vi "Raycaster_DrawSubBuffer.vi"(5 "Sub Buffer":u8, 7 "Num Columns":i16=100, 8 "Wall Height In":i16[](array[numeric]), 9 "Buffer In":u8[](array[numeric]), 10 "Game State":T1, 11 "Camera X":fxp<+/-,32,16>[](array[numeric])) -> (0 "Wall Height Out":i16[](array[numeric]), 1 "Buffer Out":u8[](array[numeric]))   [LabVIEW 2020]
uses:
  Controls/Game_State.ctl
  Controls/Player_LocationInfo.ctl
  Controls/Player_LocationInfoAxis.ctl
  Controls/Map_Position.ctl
  Controls/Raycaster_DDACalcs.ctl
  Controls/Raycaster_WallColumnAxis.ctl
  Math_FXPtoI16.vi
  Math_Multiply_FXP.vi
  Math_Add_FXP.vi
  Math_Reciprocal.vi
  Math_Subtract_FXP.vi
  Globals/MAP_DIM.vi
  Map_ReadValue.vi
  Math_Divide_FXP.vi
  Globals/HEIGHT_DIV_2.vi
  Map_GetMaps.vi
  Globals/FGV_TileVisible.vi
  <vilib>/Utility/file.llb/Application Directory.vi
  <vilib>/rvi/DataTransferAndStorage/Container/XNode/niFpgaContainer.xnode
  <vilib>/rvi/Memory/Memory_Emulation/nirvimemoryEmulation.vi
  <vilib>/rvi/Memory/Memory_Emulation/nirvimemoryFastEmulation.vi
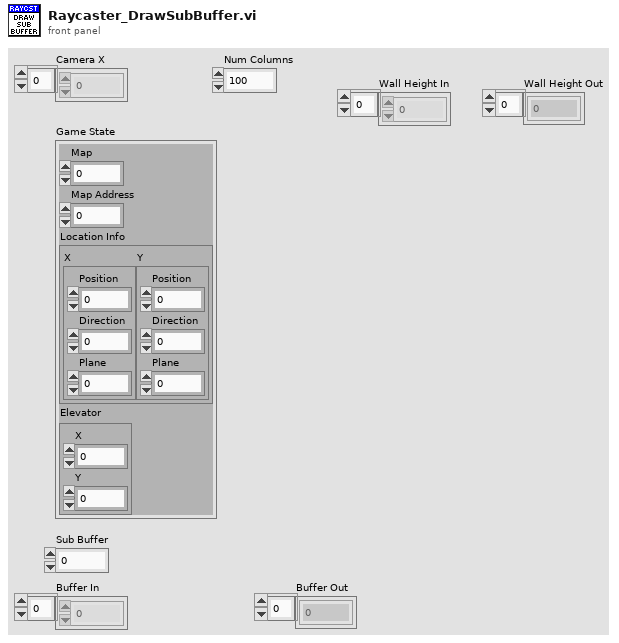
[diagram p1: front panel]
types:
  T1 = typedef "Game_State.ctl" = cluster{"Map":u8, "Map Address":u32, "Location Info":T2, "Elevator":T4}
  T2 = typedef "Player_LocationInfo.ctl" = cluster{"X":T3, "Y":T3}
  T3 = typedef "Player_LocationInfoAxis.ctl" = cluster{"Position":fxp<+/-,32,16>, "Direction":fxp<+/-,32,16>, "Plane":fxp<+/-,32,16>}
  T4 = typedef "Map_Position.ctl" = cluster{"X":fxp<+/-,32,16>, "Y":fxp<+/-,32,16>}
  T5 = typedef "Raycaster_DDACalcs.ctl" = cluster{"X":T6, "Y":T6, "Side":u8, "Perp Wall Distance":fxp<+/-,32,16>, "Wall Collision":u8}
  T6 = typedef "Raycaster_WallColumnAxis.ctl" = cluster{"Ray Direction":fxp<+/-,32,16>, "Side Distance":fxp<+/-,32,16>, "Delta Distance":fxp<+/-,32,16>, "Step":i16, "Map":i16}
  T7 = typedef "Raycaster_ScreenCalcs.ctl" = cluster{"Length":i16, "Pixel Start":i16, "Pixel End":i16, "Draw Start":i16}
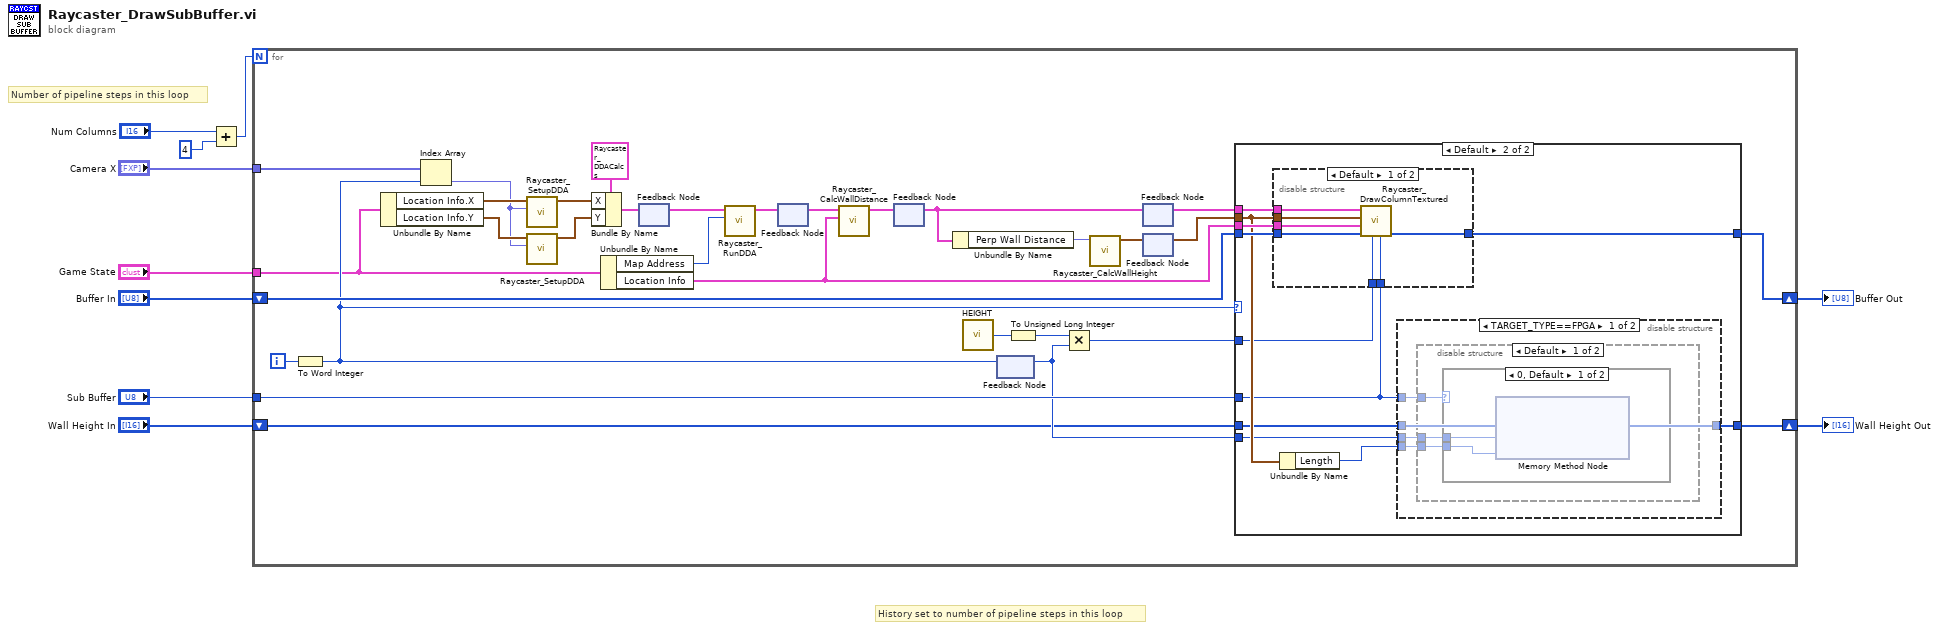
[diagram p0: block diagram]
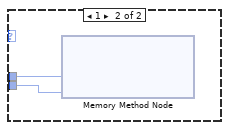
[diagram p3: hidden frame]
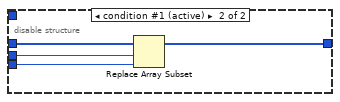
[diagram p5: hidden frame]
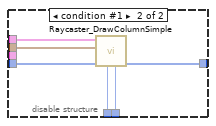
[diagram p6: hidden frame]
diagram:
  # "History set to number of pipeline steps in this loop"
  # "Number of pipeline steps in this loop"
  n1 = Add(x="Num Columns", y=i16 4) -> (x+y=w6:i16)
  n2 = for {
    N: w6 -> [_]
    tunnel: "Camera X" -> [w24]
    tunnel: "Game State" -> [w19]
    shift-right: [w26] -> w7
    shift-left: "Buffer In" -> [w27]
    tunnel: "Sub Buffer" -> [w21]
    shift-right: [w14] -> w1
    shift-left: "Wall Height In" -> [w15]
    i -> [w36]
    n3 = To Word Integer(number=w36) -> (16bit integer=w23:i16)
    n4 = Unbundle By Name(w19) -> ("Location Info.X"=w41:T3, "Location Info.Y"=w40:T3)
    n5 = Index Array(array=w24, index=w23) -> (element=w25:fxp<+/-,32,16>)
    n6 = call "Raycaster_SetupDDA.vi"("Camera X"=w25, "Location Info (Axis)"=w41) -> ("Wall Column (Axis)"=w38:T6)  [unwired: 9 in]
    n7 = call "Raycaster_SetupDDA.vi"("Camera X"=w25, "Location Info (Axis)"=w40) -> ("Wall Column (Axis)"=w37:T6)  [unwired: 9 in]
    n8 = Bundle By Name(cluster=T5 {"X"={"Ray Direction"=0.0, "Side Distance"=0.0, "Delta Distance"=0.0, "Step"=0, "Map"=0}, "Y"={"Ray Direction"=0.0, "Side Distance"=0.0, "Delta Distance"=0.0, "Step"=0, "Map"=0}, "Side"=0, "Perp Wall Distance"=0.0, "Wall Collision"=0} ("DDA Calculation"), "X"=w38, "Y"=w37) -> (w35:T5)
    n9 = Unbundle By Name(w19) -> ("Map Address"=w18:u32, "Location Info"=w17:T2)
    n10 = feedback-in #1(w35) -> ()
    n11 = feedback #1() -> (w34:T5)  [unwired: 1 in]
    n12 = call "Raycaster_RunDDA.vi"("Map Address"=w18, "DDA Calculation In"=w34) -> ("DDA Calculation Out"=w33:T5)  [unwired: 9 in]
    n13 = feedback-in #2(w33) -> ()
    n14 = feedback #2() -> (w32:T5)  [unwired: 1 in]
    n15 = call "Raycaster_CalcWallDistance.vi"("Location Info"=w17, "DDA Calculation In"=w32) -> ("DDA Calculation Out"=w31:T5)  [unwired: 9 in]
    n16 = feedback-in #3(w31) -> ()
    n17 = feedback #3() -> (w11:T5)  [unwired: 1 in]
    n18 = Unbundle By Name(w11) -> ("Perp Wall Distance"=w12:fxp<+/-,32,16>)
    n19 = call "HEIGHT.vi"() -> ("HEIGHT"=w30:i16)
    n20 = feedback-in #4(w23) -> ()
    n21 = feedback #4() -> (w16:i16)  [unwired: 1 in]
    n22 = To Unsigned Long Integer(number=w30) -> (unsigned 32bit integer=w29:u32)
    n23 = Multiply(x=w29, y=w16) -> (x*y=w22:u32)
    n24 = call "Raycaster_CalcWallHeight.vi"("Wall Distance"=w12) -> ("Height Calcs"=w13:T7)  [unwired: 10 in]
    n25 = feedback-in #5(w11) -> ()
    n26 = feedback #5() -> (w28:T5)  [unwired: 1 in]
    n27 = feedback #6() -> (w20:T7)  [unwired: 1 in]
    n28 = feedback-in #6(w13) -> ()
    n29 = case shown="Default" w23 {
      tunnel: w17 -> [_ w52]
      tunnel: w28 -> [_ w51]
      tunnel: w22 -> [_ w47]
      tunnel: w27 -> [w43 w54]
      tunnel: [w43 w53] -> w26
      tunnel: w21 -> [_ w49]
      tunnel: w20 -> [_ w50]
      tunnel: w16 -> [_ w46]
      tunnel: w15 -> [w42 w45]
      tunnel: [w42 w44] -> w14
      frame 0..3 {
        # "Don't calc / draw column, as pipelined data not yet ready,\n\n#TODO\nUpdate this case if number pipeline steps changes,"
      }
      frame Default {
        n30 = disable-structure shown="Default" {
          disable-tunnel: w51 -> [w76 w82]
          disable-tunnel: w54 -> [w75 w80]
          disable-tunnel: [w74 w79] -> w53
          disable-tunnel: w47 -> [w73 w78]
          disable-tunnel: w49 -> [w72 w77]
          disable-tunnel: w52 -> [w71 _]
          disable-tunnel: w50 -> [w70 w81]
          frame condition #0 (active) {
            n31 = call "Raycaster_DrawColumnTextured.vi"("Sub Buffer"=w72, "column"=w73, "Buffer In"=w75, "Location Info"=w71, "Column Calcs"=w70, "DDA Calculation In"=w76) -> ("Buffer Out"=w74:u8[])  [unwired: 5 in]
          }
          frame condition #1 {
            n32 = call "Raycaster_DrawColumnSimple.vi"("Sub Buffer"=w77, "column"=w78, "Buffer In"=w80, "Column Calcs"=w81, "DDA Calculation In"=w82) -> ("Buffer Out"=w79:u8[])  [unwired: 6 in]
          }
        }
        n33 = Unbundle By Name(w50) -> ("Length"=w48:i16)
        n34 = disable-structure shown="TARGET_TYPE==FPGA" {
          disable-tunnel: w48 -> [w55 w66]
          disable-tunnel: w46 -> [w56 w69]
          disable-tunnel: w45 -> [w58 w68]
          disable-tunnel: [w58 w67] -> w44
          disable-tunnel: w49 -> [w57 _]
          frame condition #0 {
            n35 = disable-structure shown="Default" {
              disable-tunnel: w57 -> [w61 _]
              disable-tunnel: w56 -> [w60 _]
              disable-tunnel: w55 -> [w59 _]
              frame condition #0 (active) {
                n36 = case shown="0, Default" w61 {
                  tunnel: w60 -> [w63 w65]
                  tunnel: w59 -> [w62 w64]
                  frame 0, Default {
                    n37 = xnode ("Memory Method Node")("Address"=w63, "Data"=w62) -> ()  [unwired: 1 in, 1 out]
                  }
                  frame 1 {
                    n38 = xnode ("Memory Method Node")("Address"=w65, "Data"=w64) -> ()  [unwired: 1 in, 1 out]
                  }
                }
              }
              frame condition #1 {
              }
            }
          }
          frame condition #1 (active) {
            n39 = Replace Array Subset(array=w68, new element=w66, index=w69) -> (w67:i16[])
          }
        }
      }
    }
  }
  "Buffer Out" <- w7
  "Wall Height Out" <- w1
